vi "s-2 dışardan alınan string değer ile diğer string değeri birleştiren pr 2018 19.vi"() -> ()   [LabVIEW 2014]
panel:
  out "String 2":string
  in  "String":string
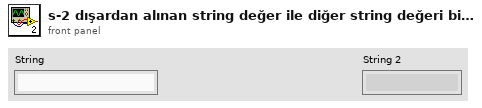
[diagram p1: front panel]
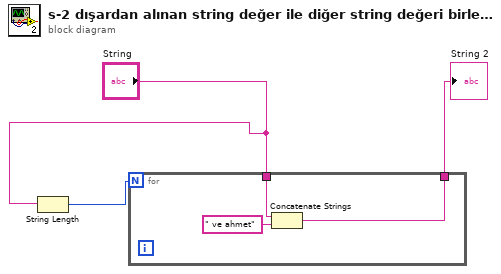
[diagram p0: block diagram]
diagram:
  n1 = String Length(string="String") -> (length=w3:i32)
  n2 = for {
    N: w3 -> [_]
    tunnel: "String" -> [w6]
    tunnel: [w4] -> w1
    n3 = Concatenate Strings(w6, " ve ahmet" ("string")) -> (w4:string)
  }
  "String 2" <- w1
